vi "Stage ReadWrite.vi"(8 "Error In":errorcluster, 10 "Hardware Configuration":T1={"XY Stage"={"COM port"="COM7", "XY stage available"=FALSE}, "DAQ FPGA"={"Ref"=refnum, "Target"="RIO0", "Clock Freq (MHz) "=200.0, "input card type"=enum."AC Card", "Samples Wait after Trigger"=5080, "AOD fill"=4900, "StartupDelay"=0, "Slip Cycle (clock cycles)"=600000, "Add Cycle"=TRUE}, "Control system"={"Ethernet opened"=FALSE, "Ethernet Port"=3, "Ctrl FPGA available"=FALSE, "Ctrl FPGA Clock (MHz)"=240.0, "Ctrl system MAC address"="", "Control system.Network adapter name"="", "AOD 1 Amplitude"=0, "AOD 2 Amplitude"=0, "AOD 3 Amplitude"=0, "AOD 4 Amplitude"=0, "AOD 5 Amplitude"=0, "AOD 6 Amplitude"=0, "Data Time Interval (ns)"=0.0, "T0 (ns)"=0.0, "Ta (ns)"=0.0}, "Encoder"={"IP address"="", "Port"=7000, "Encoder available"=FALSE, "Wheel radius (cm)"=16.0}, "DAQmx Chan"={"Pockels AO"="", "Hard shutter AO"="", "PMT AOs"="", "Power meter AI"=""}, "Computer MAC address"="", "Cam VidRec"={"DO flag-Video record"="", "DO flag-Trial start"="", "VidRec available"=FALSE}, "Externalise Triggers"=FALSE, "MC Supported"=FALSE, "Laser wavelength (nm)"=920.0} {"Laser wavelength (nm)" min=800.0 max=1080.0 step=1.0; "Encoder"."Wheel radius (cm)" format="%#_13g"; "Control system"."Ctrl FPGA Clock (MHz)" min=80.0 max=500.0 step=1.0; "Control system"."Data Time Interval (ns)" min=0.0 max=2048.0 step=1.0; "Control system"."Ta (ns)" min=0.0 max=2048.0 step=1.0; "Control system"."T0 (ns)" min=0.0 max=2048.0 step=1.0; "Control system"."AOD 6 Amplitude" min=0 max=2048 step=1; "Control system"."AOD 5 Amplitude" min=0 max=2048 step=1; "Control system"."AOD 4 Amplitude" min=0 max=2048 step=1; "Control system"."AOD 3 Amplitude" min=0 max=2048 step=1; "Control system"."AOD 2 Amplitude" min=0 max=2048 step=1; "Control system"."AOD 1 Amplitude" min=0 max=2048 step=1}, 11 "Stage Notifier":refnum<notifier>) -> (0 "Error Out":errorcluster, 3 "Stage XYZ Position":cluster{"X":sgl, "Y":sgl, "Z":sgl})   [LabVIEW 2017]
uses:
  Typedefs/Sys Configuration.ctl
  RIG-SPECIFIC FILES/FPGA Refs/FPGA Ref.ctl
  <vilib>/userdefined/High Color/nirio_resource_hc.ctl
  Typedefs/XY Stage config cluster.ctl
  Typedefs/DAQ FPGA config cluster.ctl
  Typedefs/DAQmx physical channels cluster.ctl
  Typedefs/CTRL system config cluster.ctl
  Typedefs/FPGA input type AC-DC.ctl
  Typedefs/Encoder config cluster.ctl
  Typedefs/Cam VidRec HW config setup cluster.ctl
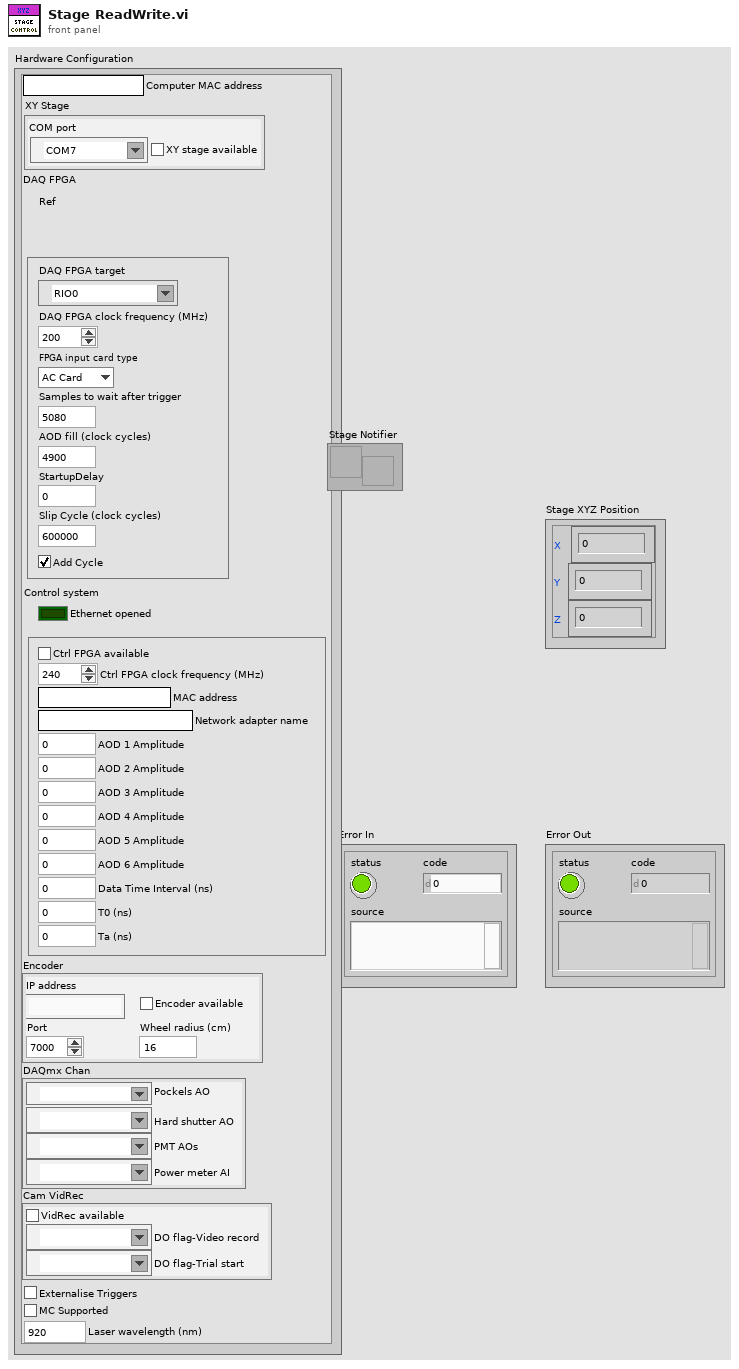
[diagram p1: front panel]
types:
  T1 = typedef "Sys Configuration.ctl" = cluster{"XY Stage":T2, "DAQ FPGA":T3, "Control system":T7, "Encoder":T8, "DAQmx Chan":T9, "Computer MAC address":string, "Cam VidRec":T10, "Externalise Triggers":bool, "MC Supported":bool, "Laser wavelength (nm)":dbl}
  T2 = typedef "XY Stage config cluster.ctl" = cluster{"COM port":refnum<visa-resource-name>, "XY stage available":bool}
  T3 = typedef "DAQ FPGA config cluster.ctl" = cluster{"Ref":T4, "Target":T5, "Clock Freq (MHz) ":dbl, "input card type":T6, "Samples Wait after Trigger":u16, "AOD fill":u16, "StartupDelay":i32, "Slip Cycle (clock cycles)":u32, "Add Cycle":bool}
  T4 = typedef "FPGA Ref.ctl" = refnum<k20>
  T5 = typedef "nirio_resource_hc.ctl" = tag
  T6 = typedef "FPGA input type AC-DC.ctl" = enum16{"AC Card", "DC Card"}
  T7 = typedef "CTRL system config cluster.ctl" = cluster{"Ethernet opened":bool, "Ethernet Port":u32, "Ctrl FPGA available":bool, "Ctrl FPGA Clock (MHz)":dbl, "Ctrl system MAC address":string, "Control system.Network adapter name":string, "AOD 1 Amplitude":i16, "AOD 2 Amplitude":i16, "AOD 3 Amplitude":i16, "AOD 4 Amplitude":i16, "AOD 5 Amplitude":i16, "AOD 6 Amplitude":i16, "Data Time Interval (ns)":dbl, "T0 (ns)":dbl, "Ta (ns)":dbl}
  T8 = typedef "Encoder config cluster.ctl" = cluster{"IP address":string, "Port":u16, "Encoder available":bool, "Wheel radius (cm)":dbl}
  T9 = typedef "DAQmx physical channels cluster.ctl" = cluster{"Pockels AO":tag, "Hard shutter AO":tag, "PMT AOs":tag, "Power meter AI":tag}
  T10 = typedef "Cam VidRec HW config setup cluster.ctl" = cluster{"DO flag-Video record":tag, "DO flag-Trial start":tag, "VidRec available":bool}
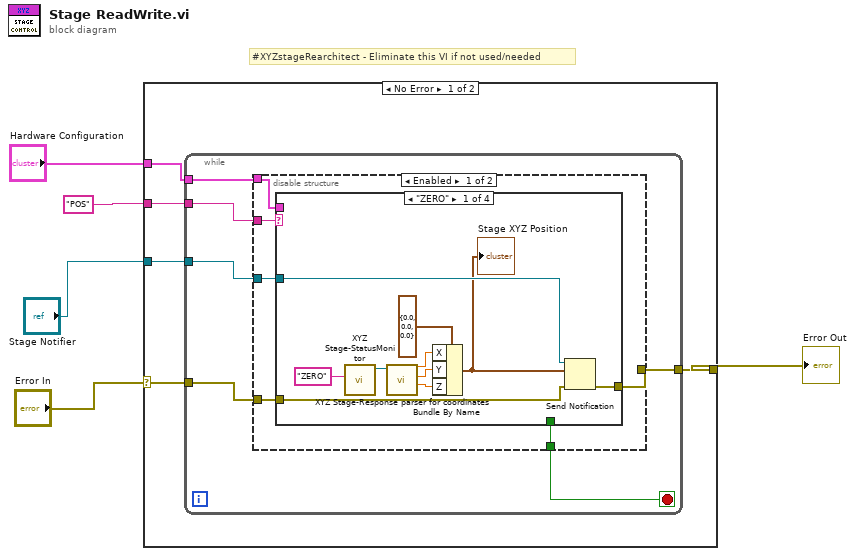
[diagram p0: block diagram]
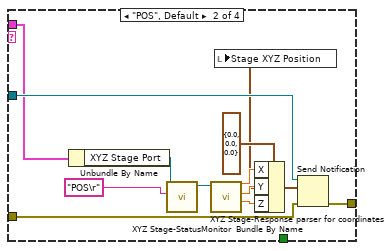
[diagram p2: hidden frame]
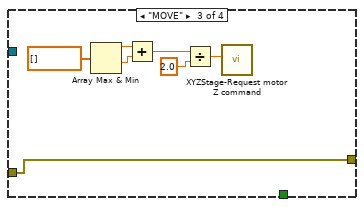
[diagram p3: hidden frame]
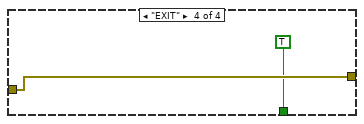
[diagram p4: hidden frame]
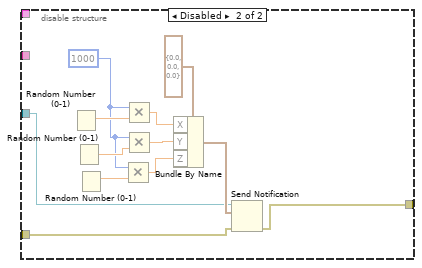
[diagram p5: hidden frame]
diagram:
  # "#XYZstageRearchitect - Eliminate this VI if not used/needed"
  n1 = case shown="No Error" "Error In" {
    selector: "Error In" -> [w8 w66]
    tunnel: [w7 w66] -> w4
    tunnel: "Hardware Configuration" -> [w6 _]
    tunnel: "Stage Notifier" -> [w10 _]
    tunnel: "POS" -> [w9 _]
    frame No Error {
      n2 = while {
        tunnel: w10 -> [w16]
        tunnel: w9 -> [w15]
        tunnel: w8 -> [w14]
        tunnel: [w13] -> w7
        tunnel: w6 -> [w11]
        stop <- w12 stop-if-true
        n3 = disable-structure shown="Enabled" {
          disable-tunnel: w16 -> [w22 w63]
          disable-tunnel: w15 -> [w21 _]
          disable-tunnel: w14 -> [w20 w62]
          disable-tunnel: [w19 w61] -> w13
          disable-tunnel: [w18 _] -> w12
          disable-tunnel: w11 -> [w17 _]
          frame Enabled {
            n4 = case shown="\"ZERO\"" w21 {
              tunnel: w22 -> [w32 w44 _ _]
              tunnel: w20 -> [w23 w38 w45 w53]
              tunnel: [w24 w37 w45 w53] -> w19
              tunnel: [_ _ _ TRUE] -> w18
              tunnel: w17 -> [_ w36 _ _]
              frame "ZERO" {
                n5 = call "XYZ Stage-StatusMonitor.vi"("string to write"="ZERO") -> ("VISA resource name out"=w30:refnum<visa-resource-name>)  [unwired: 7 in, 3 out]
                n6 = call "XYZ Stage-Response parser for coordinates.vi"("Filtered response string (no CR)"=w30) -> ("Z"=w25:sgl, "Y"=w26:sgl, "X"=w27:sgl)  [unwired: 8 in]
                n7 = Bundle By Name(cluster=cluster{"X":sgl, "Y":sgl, "Z":sgl} {"X"=0.0, "Y"=0.0, "Z"=0.0} ("Stage XYZ Position"), "X"=w27, "Y"=w26, "Z"=w25) -> (w28:cluster{"X":sgl, "Y":sgl, "Z":sgl})
                "Stage XYZ Position" <- w28
                n8 = Send Notification(notification=w28, notifier=w32, error in (no error)=w23) -> (error out=w24:errorcluster)  [unwired: 1 out]
              }
              frame "POS", Default {
                n9 = Unbundle By Name(w36) -> ("XYZ Stage Port"=w35:refnum<visa-resource-name>)
                n10 = call "XYZ Stage-StatusMonitor.vi"("string to write"="POS\r", "VISA resource name"=w35) -> ("VISA resource name out"=w43:refnum<visa-resource-name>)  [unwired: 6 in, 3 out]
                n11 = call "XYZ Stage-Response parser for coordinates.vi"("Filtered response string (no CR)"=w43) -> ("Z"=w39:sgl, "Y"=w40:sgl, "X"=w41:sgl)  [unwired: 8 in]
                n12 = Bundle By Name(cluster=cluster{"X":sgl, "Y":sgl, "Z":sgl} {"X"=0.0, "Y"=0.0, "Z"=0.0} ("Stage XYZ Position"), "X"=w41, "Y"=w40, "Z"=w39) -> (w34:cluster{"X":sgl, "Y":sgl, "Z":sgl})
                n13 = local write "Stage XYZ Position"(w34) -> ()
                n14 = Send Notification(notification=w34, notifier=w44, error in (no error)=w38) -> (error out=w37:errorcluster)  [unwired: 1 out]
              }
              frame "MOVE" {
                n15 = Array Max & Min(array=dbl[] []) -> (max value=w51:dbl, min value=w50:dbl)  [unwired: 2 out]
                n16 = Add(x=w51, y=w50) -> (x+y=w48:dbl)
                n17 = Divide(x=w48, y=2.0) -> (x/y=w49:dbl)
                n18 = call "XYZStage-Request motor Z command.vi"("Motor Z"=w49) -> ()  [unwired: 8 in, 3 out]
              }
              frame "EXIT" {
              }
            }
          }
          frame Disabled {
            w54 = 1000
            n19 = Random Number (0-1)() -> (number: 0 to 1=w60:dbl)
            n20 = Random Number (0-1)() -> (number: 0 to 1=w55:dbl)
            n21 = Random Number (0-1)() -> (number: 0 to 1=w57:dbl)
            n22 = Multiply(x=w54, y=w57) -> (x*y=w58:dbl)
            n23 = Multiply(x=w54, y=w60) -> (x*y=w59:dbl)
            n24 = Multiply(x=w54, y=w55) -> (x*y=w56:dbl)
            n25 = Bundle By Name(cluster=cluster{"X":sgl, "Y":sgl, "Z":sgl} {"X"=0.0, "Y"=0.0, "Z"=0.0} ("Stage XYZ Position"), "X"=w59, "Y"=w56, "Z"=w58) -> (w64:cluster{"X":sgl, "Y":sgl, "Z":sgl})
            n26 = Send Notification(notification=w64, notifier=w63, error in (no error)=w62) -> (error out=w61:errorcluster)  [unwired: 1 out]
          }
        }
      }
    }
    frame Error {
    }
  }
  "Error Out" <- w4
